vi "Read Registry Value.vi"   [LabVIEW 2012]
doc: "Reads data and the data type from value. If the key or value does not exist, the VI returns the default value."
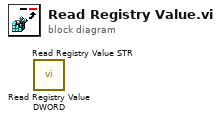
[diagram p0: block diagram]
diagram:
  n1 = call "Read Registry Value DWORD.vi"() -> ()  [unwired: 8 in, 4 out]
  n2 = call "Read Registry Value STR.vi"() -> ()  [unwired: 8 in, 4 out]
